vi "FTW-TestSupport-Actor-EchoServer.vi"(0 "Actor Instance Configuration":string="{\n  \"Identity\": \"ActorName\",\n  \"InboxAddress\": \"tcp://127.0.0.1:*\",\n  \"SupervisorAddress\": \"\",\n  \"DebugEnableInboxLogging\": false,\n  \"DebugEnableJobLogging\": false,\n  \"DebugShowPanel\": false\n}", 5 "Deadline (maximum actor lifetime)":i32=5000 format="%dmsec", 11 "ErrorIn":errorcluster) -> (15 "Error":errorcluster)   [LabVIEW 2015]
uses:
  src/actor/instance/FTW-Actor-Instance.lvclass
  src/json/FTW-JSON-Type.ctl
  codegen/xnode/FTW-JSON-Fetch.xnode
  src/core/type/FTW-Type-JSON.ctl
  lib/FTW-KernelFilepath.vi
  src/json/core/FTW-JSON-Core-LibraryReturnValue.vi
  src/error/FTW-ERR-ThrowInvalidReferenceError.vi
  src/json/core/FTW-JSON-Core-Type.ctl
  src/json/core/FTW-JSON-Core-ElementType.vi
panel:
  # "Inputs"
  # "Outputs"
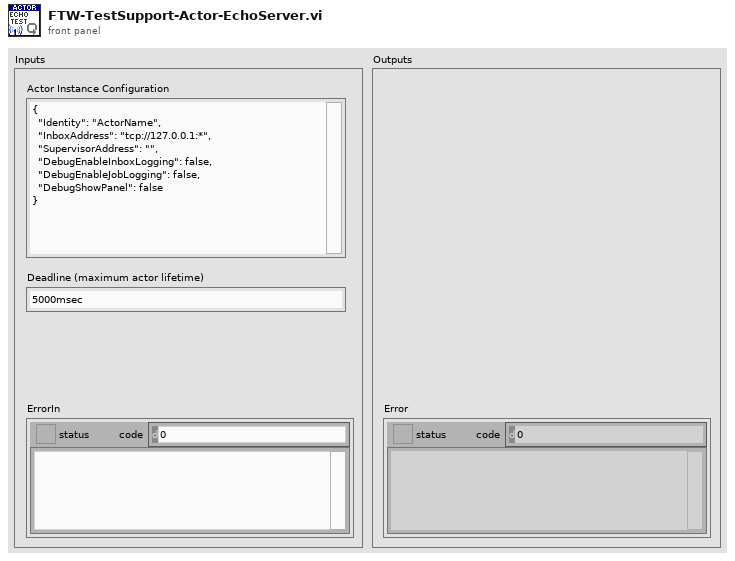
[diagram p1: front panel]
types:
  T1 = cluster{"Incoming Request":refnum<event-registration>}
  T2 = typedef "FTW-JSON-Core-Type.ctl" = enum8{"Object", "Array", "String", "Integer", "Floating Point", "true", "false", "null", "undefined"}
  T3 = typedef "FTW-Type-JSON.ctl" = refnum<data-value>
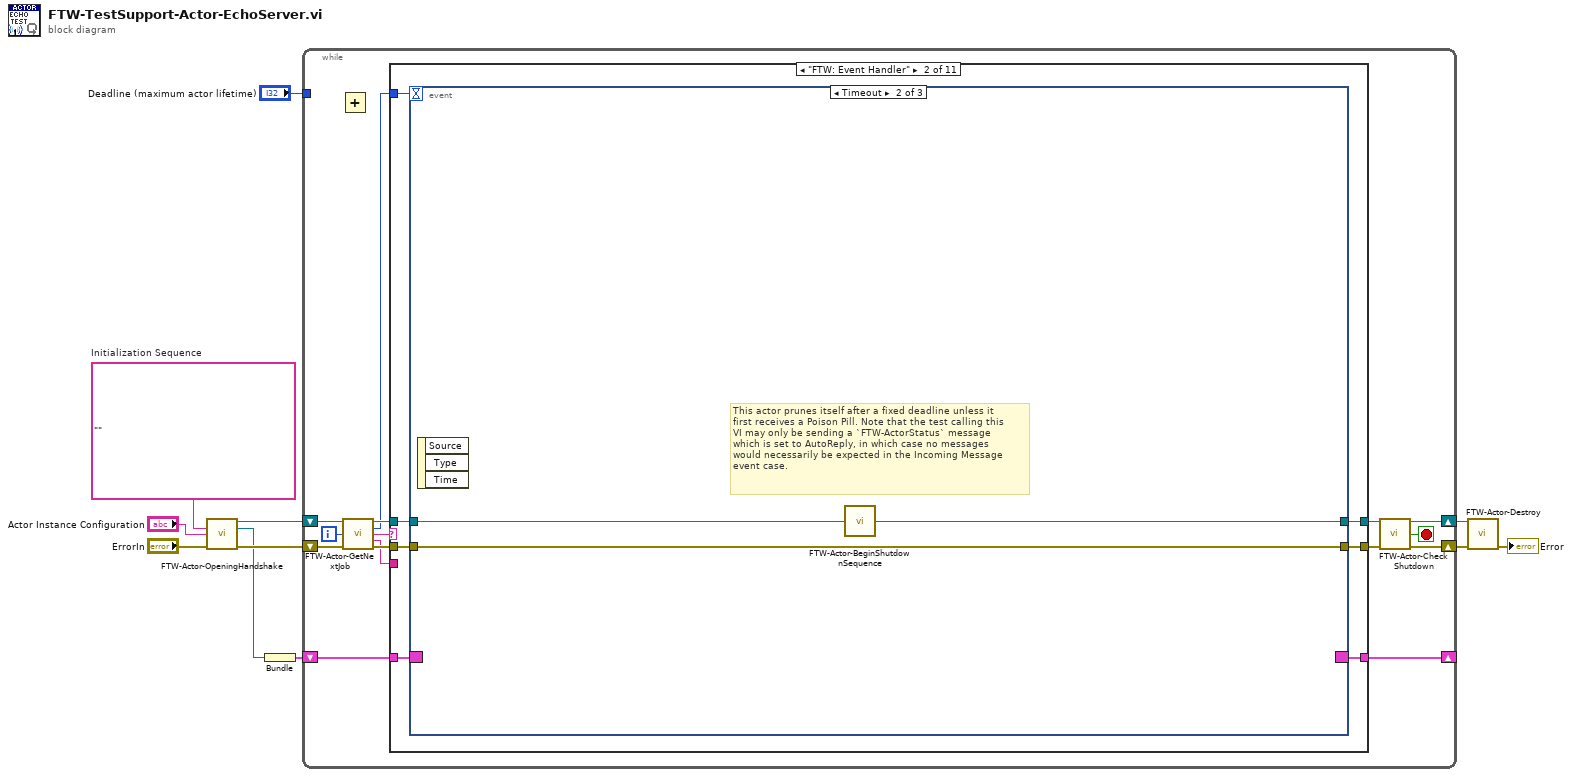
[diagram p0: block diagram]
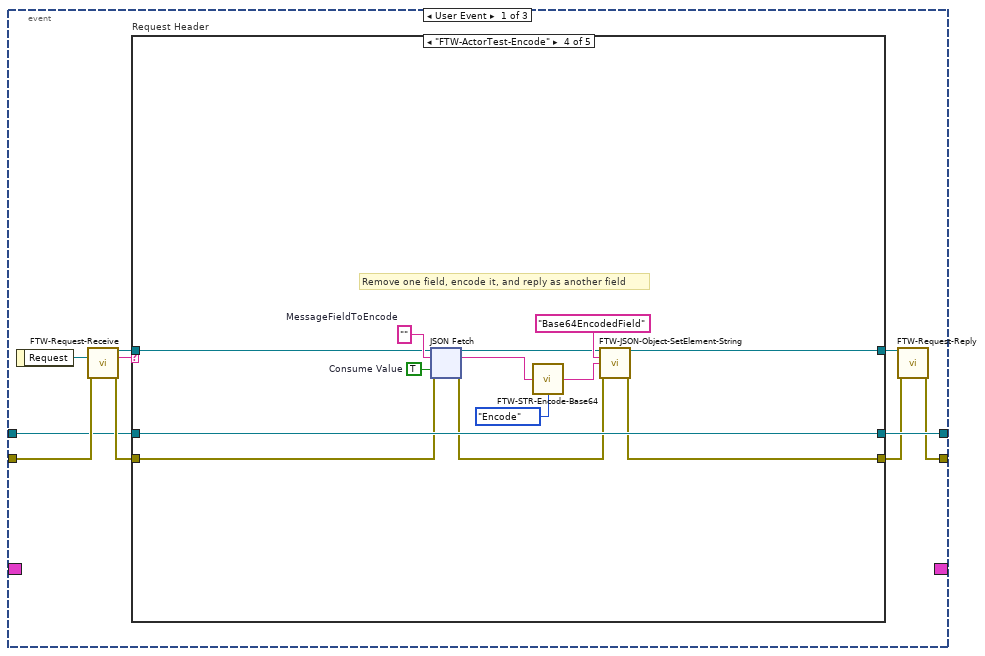
[diagram p3: hidden frame]
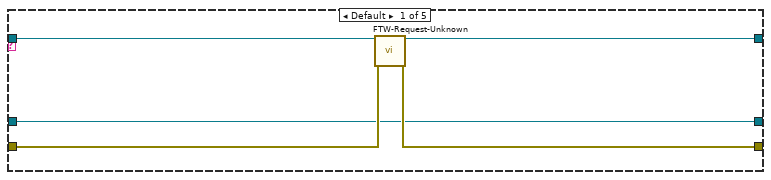
[diagram p4: hidden frame]
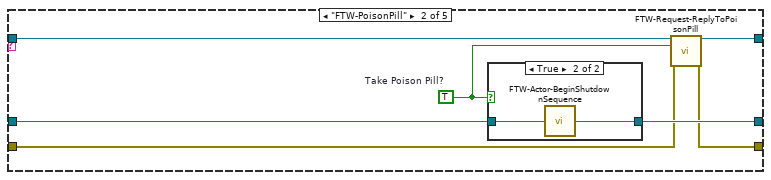
[diagram p5: hidden frame]
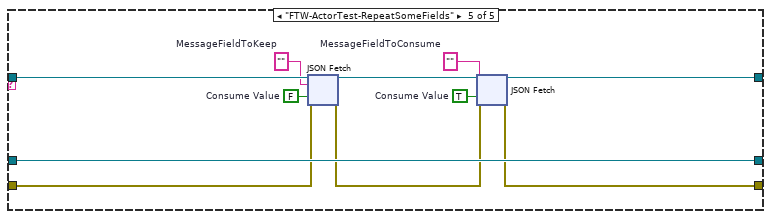
[diagram p8: hidden frame]
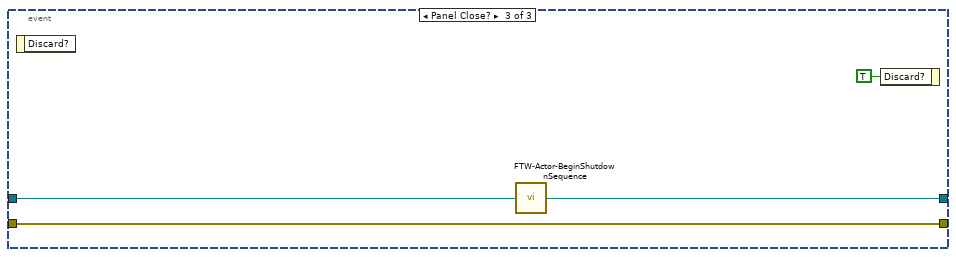
[diagram p9: hidden frame]
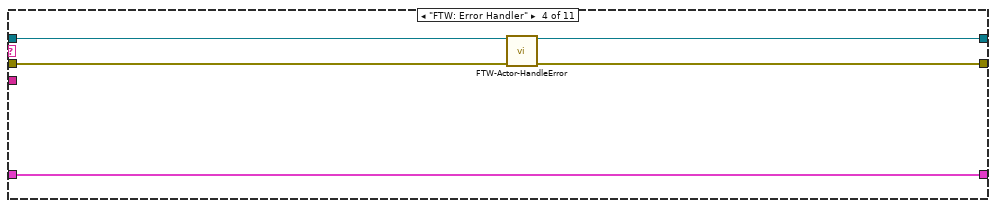
[diagram p11: hidden frame]
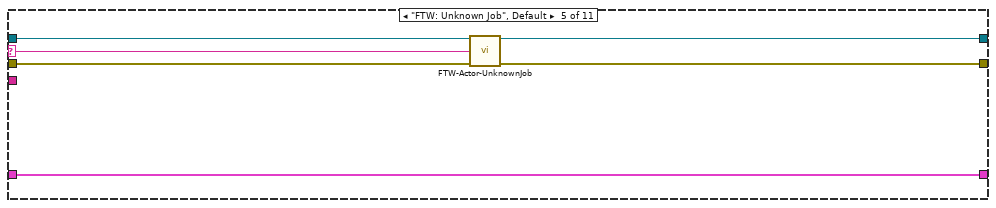
[diagram p12: hidden frame]
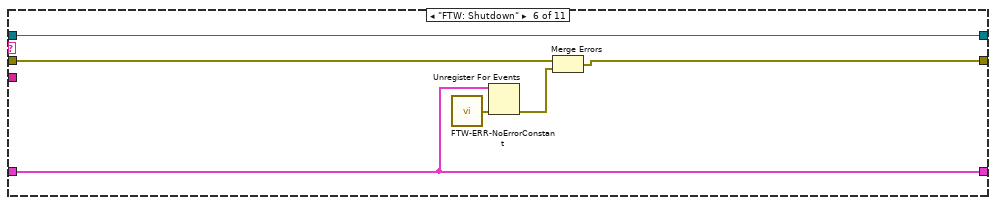
[diagram p13: hidden frame]
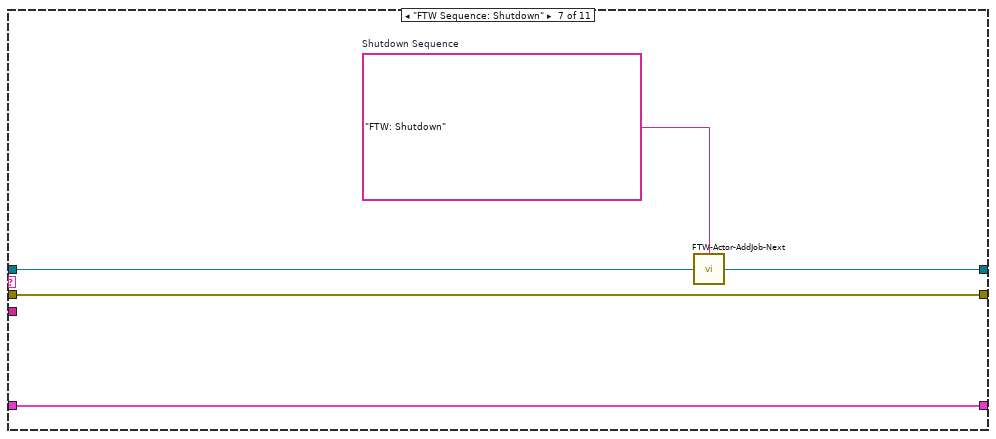
[diagram p14: hidden frame]
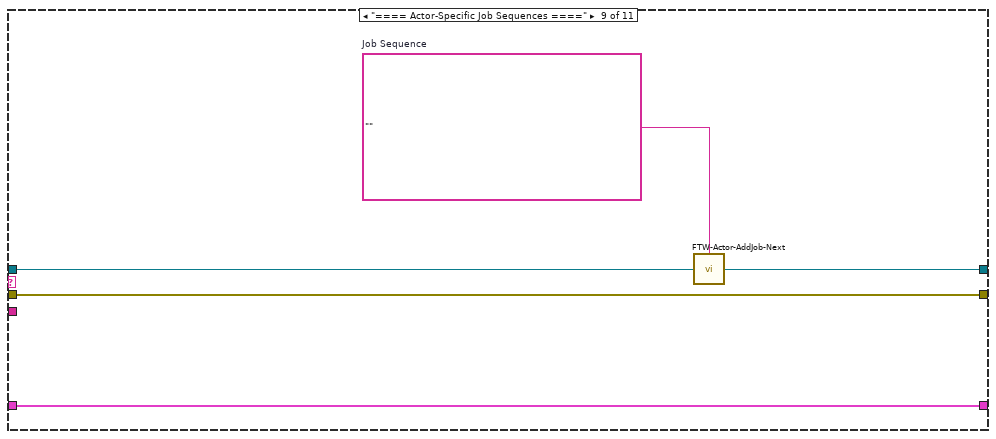
[diagram p16: hidden frame]
diagram:
  w6 = ""  # Initialization Sequence
  n1 = call "FTW-Actor-OpeningHandshake.vi"("Initialization Job Sequence"=w6, "Actor Instance Configuration"="Actor Instance Configuration", "error in"="ErrorIn") -> ("FTW Actor Instance"=w11:refnum<class "FTW-Actor-Instance.lvclass">, "Incoming Request"=w2:refnum<event-registration>, "error out"=w7:errorcluster)  [unwired: 10 in]
  n2 = Bundle("Incoming Request"=w2) -> (w1:T1)  [unwired: 1 in]
  n3 = while {
    shift-right: [w16] -> w9
    shift-left: w7 -> [w23]
    shift-right: [w14] -> _
    shift-left: w1 -> [w26]
    shift-right: [w18] -> w10
    shift-left: w11 -> [w25]
    tunnel: "Deadline (maximum actor lifetime)" -> [_]
    i -> [w15]
    stop <- w12 stop-if-true
    n4 = Add() -> ()  [unwired: 2 in, 1 out]
    n5 = call "FTW-Actor-GetNextJob.vi"("FTW Actor Instance"=w25, "Jobs Performed"=w15, "error in"=w23) -> ("FTW Actor Instance out"=w24:refnum<class "FTW-Actor-Instance.lvclass">, "Event Structure Timeout"=w13:i32, "Job Name"=w21:string, "Job Data"=w20:string, "error out"=w22:errorcluster)  [unwired: 8 in]
    n6 = case shown="\"FTW: Event Handler\"" w21 {
      selector: w21 -> [_ _ _ _ w236 _ _ _ _ _ _]
      tunnel: [w28 w36 w228 w231 w239 w246 w251 w254 w259 w263 w266] -> w17
      tunnel: w22 -> [w28 w35 w228 w233 w240 w247 w251 w254 w259 w263 w266]
      tunnel: w26 -> [w29 w31 w230 w235 w241 w243 w252 w255 w260 w262 w265]
      tunnel: [w29 w34 w230 w235 w241 w243 w252 w255 w260 w262 w265] -> w14
      tunnel: w20 -> [_ _ _ _ _ _ _ _ _ _ _]
      tunnel: [w27 w33 w229 w232 w237 w244 w249 w253 w257 w261 w264] -> w19
      tunnel: w24 -> [w27 w32 w229 w234 w238 w244 w250 w253 w258 w261 w264]
      tunnel: w13 -> [_ w30 _ _ _ _ _ _ _ _ _]
      frame "==== Featherweight Framework Jobs ====" {
      }
      frame "FTW: Event Handler" {
        n7 = event shown="[1] Timeout" {
          selector: w31 -> [_ _ _]
          dyn-events: [_ _ _] -> w34
          timeout: w30 -> [_ _ _]
          tunnel: [w40 w223 w226] -> w36
          tunnel: w35 -> [w45 w223 w226]
          tunnel: [w44 w221 w224] -> w33
          tunnel: w32 -> [w43 w222 w225]
          event User Event {
            n8 = event-data() -> ("Request"=w37:refnum<queue>)  [unwired: 1 in]
            n9 = call "FTW-Request-Receive.vi"("MessagePipe"=w37, "error in"=w45) -> ("Request"=w41:T3, "Request Header"=w42:string, "error out"=w46:errorcluster)  [unwired: 11 in]
            n10 = case "Request Header" shown="\"FTW-ActorTest-Encode\"" w42 {
              tunnel: [w50 w53 w62 w75 w122] -> w39
              tunnel: w46 -> [w51 w54 w62 w70 w128]
              tunnel: [w48 w58 w64 w77 w132] -> w44
              tunnel: w43 -> [w48 w57 w64 w77 w132]
              tunnel: w41 -> [w49 w56 w63 w65 w131]
              tunnel: [w47 w55 w63 w76 w123] -> w38
              frame Default {
                n11 = call "FTW-Request-Unknown.vi"("Request"=w49, "error in"=w51) -> ("Request out"=w47:T3, "error out"=w50:errorcluster)  [unwired: 12 in]
              }
              frame "FTW-PoisonPill" {
                w52 = TRUE  # Take Poison Pill?
                n12 = case shown="True" w52 {
                  tunnel: [w59 w61] -> w58
                  tunnel: w57 -> [w59 w60]
                  frame False {
                  }
                  frame True {
                    n13 = call "FTW-Actor-BeginShutdownSequence.vi"("FTW Actor Instance"=w60) -> ("FTW Actor Instance out"=w61:refnum<class "FTW-Actor-Instance.lvclass">)  [unwired: 3 in]
                  }
                }
                n14 = call "FTW-Request-ReplyToPoisonPill.vi"("Poison Pill Request"=w56, "Shutting Down?"=w52, "error in"=w54) -> ("Poison Pill Response"=w55:T3, "error out"=w53:errorcluster)  [unwired: 11 in]
              }
              frame "FTW-ActorTest-RepeatVerbatim" {
                # "Repeat the message exactly as it was sent"
              }
              frame "FTW-ActorTest-Encode" {
                w67 = ""  # MessageFieldToEncode
                w71 = TRUE  # Consume Value
                # "Remove one field, encode it, and reply as another field"
                n15 = xnode "JSON Fetch"("JSON"=w65, "Element Type and Default Value"=w67, "Consume Element"=w71, "error in"=w70) -> ("JSON out"=w66:T3, "Value"=w69:string, "error out"=w68:errorcluster)  [unwired: 1 in, 1 out]
                n16 = call "FTW-STR-Encode-Base64.vi"("Input"=w69, "Direction"=enum16{"Encode", "Decode"}."Encode") -> ("Output"=w74:string)
                n17 = call "FTW-JSON-Object-SetElement-String.vi"("JSON"=w66, "Key"="Base64EncodedField", "Value"=w74, "error in"=w68) -> ("JSON out"=w76:T3, "error out"=w75:errorcluster)  [unwired: 10 in]
              }
              frame "FTW-ActorTest-RepeatSomeFields" {
                w126 = ""  # MessageFieldToConsume
                w127 = TRUE  # Consume Value
                w130 = ""  # MessageFieldToKeep
                w129 = FALSE  # Consume Value
                n18 = xnode "JSON Fetch"("JSON"=w131, "Element Type and Default Value"=w130, "Consume Element"=w129, "error in"=w128) -> ("JSON out"=w124:T3, "error out"=w125:errorcluster)  [unwired: 1 in, 2 out]
                n19 = xnode "JSON Fetch"("JSON"=w124, "Element Type and Default Value"=w126, "Consume Element"=w127, "error in"=w125) -> ("JSON out"=w123:T3, "error out"=w122:errorcluster)  [unwired: 1 in, 2 out]
              }
            }
            n20 = call "FTW-Request-Reply.vi"("Request"=w38, "error in"=w39) -> ("error out"=w40:errorcluster)  [unwired: 13 in]
          }
          event Timeout {
            # "This actor prunes itself after a fixed deadline unless it\nfirst receives a Poison Pill. Note that the test calling this\nVI may only be sending a `FTW-ActorStatus` message\nwhich is set to AutoReply, in which case no messages\nwould necessarily be expected in the Incoming Message\nevent case."
            n21 = event-data() -> ()  [unwired: 1 in, 3 out]
            n22 = call "FTW-Actor-BeginShutdownSequence.vi"("FTW Actor Instance"=w222) -> ("FTW Actor Instance out"=w221:refnum<class "FTW-Actor-Instance.lvclass">)  [unwired: 3 in]
          }
          event Panel Close? {
            n23 = event-data() -> ()  [unwired: 1 in, 1 out]
            n24 = call "FTW-Actor-BeginShutdownSequence.vi"("FTW Actor Instance"=w225) -> ("FTW Actor Instance out"=w224:refnum<class "FTW-Actor-Instance.lvclass">)  [unwired: 3 in]
            n25 = event-data("Discard?"=TRUE) -> ()  [unwired: 1 in, 1 out]
          }
        }
      }
      frame "FTW: Failure to Launch" {
      }
      frame "FTW: Error Handler" {
        n26 = call "FTW-Actor-HandleError.vi"("FTW Actor Instance"=w234, "error in"=w233) -> ("FTW Actor Instance out"=w232:refnum<class "FTW-Actor-Instance.lvclass">, "error out"=w231:errorcluster)  [unwired: 11 in, 1 out]
      }
      frame "FTW: Unknown Job", Default {
        n27 = call "FTW-Actor-UnknownJob.vi"("FTW Actor Instance"=w238, "Unknown Job"=w236, "error in"=w240) -> ("FTW Actor Instance out"=w237:refnum<class "FTW-Actor-Instance.lvclass">, "error out"=w239:errorcluster)  [unwired: 11 in]
      }
      frame "FTW: Shutdown" {
        n28 = call "FTW-ERR-NoErrorConstant.vi"() -> ("no error"=w242:errorcluster)
        n29 = Unregister For Events(event registration refnum=w243, error in=w242) -> (error out=w245:errorcluster)
        n30 = Merge Errors(w247, w245) -> (w246:errorcluster)
      }
      frame "FTW Sequence: Shutdown" {
        w248 = "FTW: Shutdown"  # Shutdown Sequence
        n31 = call "FTW-Actor-AddJob-Next.vi"("Add Next in Job Queue"=w248, "FTW Actor Instance"=w250) -> ("FTW Actor Instance out"=w249:refnum<class "FTW-Actor-Instance.lvclass">)  [unwired: 2 in]
      }
      frame "==== Actor-Specific Static Dependencies ====" {
      }
      frame "==== Actor-Specific Job Sequences ====" {
        w256 = ""  # Job Sequence
        n32 = call "FTW-Actor-AddJob-Next.vi"("Add Next in Job Queue"=w256, "FTW Actor Instance"=w258) -> ("FTW Actor Instance out"=w257:refnum<class "FTW-Actor-Instance.lvclass">)  [unwired: 2 in]
      }
      frame "==== Actor-Specific Jobs ====" {
      }
      frame "ActorName: Job Template" {
      }
    }
    n33 = call "FTW-Actor-CheckShutdown.vi"("FTW Actor Instance"=w19, "error in"=w17) -> ("FTW Actor Instance out"=w18:refnum<class "FTW-Actor-Instance.lvclass">, "Shutdown?"=w12:bool, "error out"=w16:errorcluster)  [unwired: 11 in]
  }
  n34 = call "FTW-Actor-Destroy.vi"("FTW Actor Instance"=w10, "error in"=w9) -> ("error out"=→"Error":errorcluster)  [unwired: 12 in, 1 out]
